vi "RSZVB Export Kit With Label.vi"(7 "File Name (\"\")":string, 8 "error in (no error)":errorcluster {"code" format="%.0x"}, 9 "Kit Label (\"\")":string, 10 "Kit Name (\"\")":string, 11 "VISA session":refnum<visa-resource-name>) -> (0 "error out":errorcluster {"code" format="%.0x"}, 3 "dup VISA session":refnum<visa-resource-name>)   [LabVIEW 2011]
doc: "Stores the data of a calibration kit to a specified file. The calibration kit is identified by its name and label. \n\nRemote-control command(s):\nMMEMory:STORe:CKIT:WLABel"
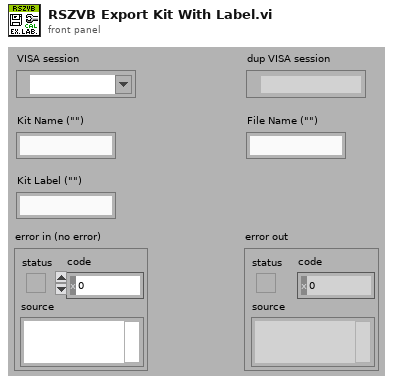
[diagram p1: front panel]
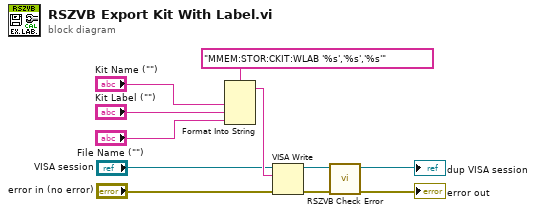
[diagram p0: block diagram]
diagram:
  n1 = Format Into String(format string="MMEM:STOR:CKIT:WLAB '%s','%s','%s'", "Kit Name (\"\")", "Kit Label (\"\")", "File Name (\"\")") -> (resulting string=w8:string)  [unwired: 2 in, 1 out]
  n2 = VISA Write(VISA resource name="VISA session", write buffer=w8, error in (no error)="error in (no error)") -> (VISA resource name out=w9:refnum<visa-resource-name>, error out=w10:errorcluster)  [unwired: 1 out]
  n3 = call "RSZVB Check Error.vi"("error in (no error)"=w10, "VISA session"=w9) -> ("error out"=→"error out":errorcluster, "dup VISA session"=→"dup VISA session":refnum<visa-resource-name>)  [unwired: 8 in]
